vi "take_i16_from_BSON_bytes.vi"(11 "BSONbytes":u8[](array[numeric])) -> (2 "restOfBytes":u8[](array[numeric]), 3 "value":i16)   [LabVIEW 2015, in "BSON_convertors_Library.lvlib"]
doc: "Created by Artem Shevelev\nLabVIEW Portal profile: http://www.labviewportal.org/memberlist.php?mode=viewprofile&u=2340\ne-mail: artem.sh@gmail.com\nshevelev.pro"
uses:
  BSON_convertors_Library.lvlib
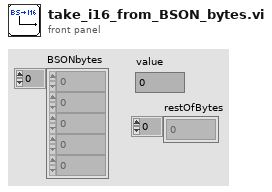
[diagram p1: front panel]
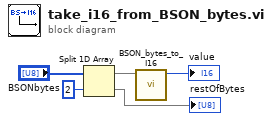
[diagram p0: block diagram]
diagram:
  n1 = Split 1D Array(array="BSONbytes", index=2) -> (first subarray=w3:u8[], second subarray=→"restOfBytes":u8[])
  n2 = call "BSON_bytes_to_I16.vi"("BSONbytes"=w3) -> ("value"=→"value":i16)  [unwired: 10 in]
